vi "get_settings_cluster.vi"(8 "error in (no error)":errorcluster, 11 "GenericPlugin in":refnum<class "StageMMS2015ASIfromScientifica.lvclass">) -> (0 "error out":errorcluster, 2 "settings cluster":variant, 3 "GenericPlugin out":refnum<class "StageMMS2015ASIfromScientifica.lvclass">)   [LabVIEW 2010, in "StageMMS2015ASIfromScientifica.lvclass"]
uses:
  StageMMS2015ASIfromScientifica.lvclass
  StageMMS2015ASIfromScientifica.lvclass/StageMMS2015ASIfromScientifica.ctl
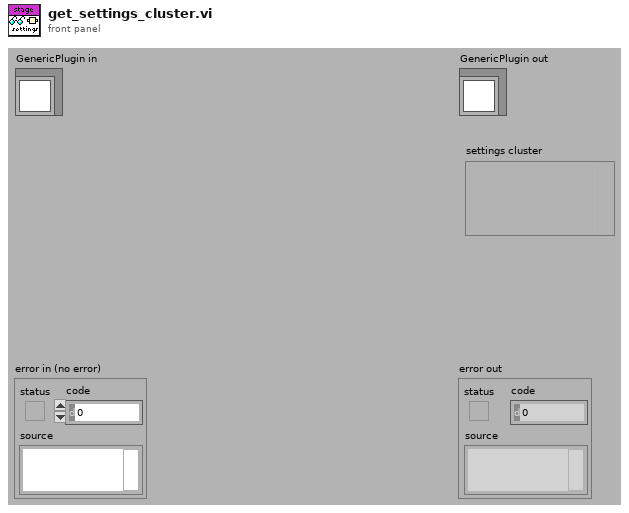
[diagram p1: front panel]
types:
  T1 = typedef "StageMMS2015ASIfromScientifica.lvclass/settings_cluster.ctl" = cluster{"empty setting thing":string}
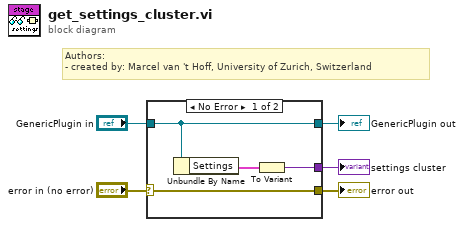
[diagram p0: block diagram]
diagram:
  # "Authors: \n- created by: Marcel van 't Hoff, University of Zurich, Switzerland"
  n1 = case shown="No Error" "error in (no error)" {
    selector: "error in (no error)" -> [w9 w11]
    tunnel: [w9 w11] -> w3
    tunnel: [w7 _] -> w2
    tunnel: "GenericPlugin in" -> [w6 w10]
    tunnel: [w6 w10] -> w1
    frame No Error {
      n2 = Unbundle By Name(w6) -> ("Settings"=w8:T1)
      n3 = To Variant(anything=w8) -> (Variant=w7:variant)
    }
    frame Error {
    }
  }
  "error out" <- w3
  "GenericPlugin out" <- w1
  "settings cluster" <- w2
